vi "Read Measurement Name.vi"(8 "error in (no error)":errorcluster, 11 "SeqAuto IEvaluation in":refnum<class "SeqAuto IEvaluation.lvclass">) -> (0 "error out":errorcluster, 2 "Measurement Name":string, 3 "SeqAuto IEvaluation out":refnum<class "SeqAuto IEvaluation.lvclass">)   [LabVIEW 2018, in "IEvaluation.lvlib" / "SeqAuto IEvaluation.lvclass"]
uses:
  SeqAuto IEvaluation.lvclass
  SeqAuto IEvaluation.lvclass/SeqAuto IEvaluation.ctl
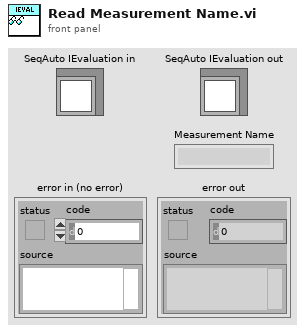
[diagram p1: front panel]
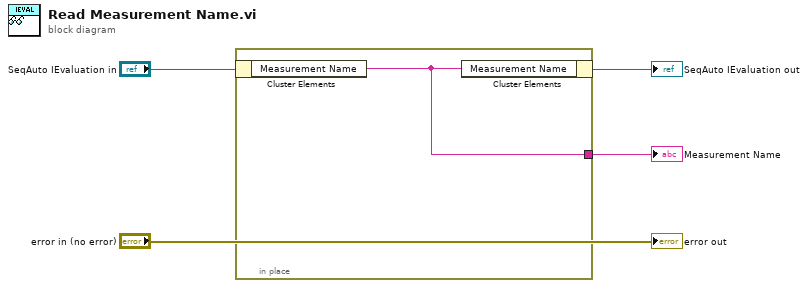
[diagram p0: block diagram]
diagram:
  n1 = in-place {
    in-place-border: [w5] -> w1
    n2 = in-place-cluster #1("SeqAuto IEvaluation in") -> ("Measurement Name"=w5:string)
    n3 = in-place-cluster #1("Measurement Name"=w5) -> (→"SeqAuto IEvaluation out":refnum<class "SeqAuto IEvaluation.lvclass">)
  }
  "Measurement Name" <- w1
  "error out" <- "error in (no error)"
